vi "Write Abstract Message Definitions.vi"(10 "Abstract Message Definitions":T1, 11 "SCADA in":refnum<class "SCADA.lvclass">) -> (3 "SCADA out":refnum<class "SCADA.lvclass">)   [LabVIEW 2015, in "SCADA Core.lvlib" / "SCADA.lvclass"]
uses:
  SCADA.lvclass
  Controls/Abstract Messages Definitions Cluster.ctl
  SCADA Abstract Messages/Simple Command Status Msg/Simple Command Status Msg.lvclass
  SCADA Abstract Messages/IED Measurement Status Msg/IED Measurement Status Msg.lvclass
  SCADA Abstract Messages/Device Action Status Msg/Device Action Status Msg.lvclass
  SCADA Abstract Messages/Device Load Status Msg/Device Load Status Msg.lvclass
  SCADA Abstract Messages/IED Setpoint Status Msg/IED Setpoint Status Msg.lvclass
  SCADA Abstract Messages/Get Device Parameter Status Msg/Get Device Parameter Status Msg.lvclass
  SCADA Abstract Messages/Set Device Parameter Status Msg/Set Device Parameter Status Msg.lvclass
  SCADA Abstract Messages/Emergency Status Msg/Emergency Status Msg.lvclass
  SCADA Abstract Messages/Black Start Status Msg/Black Start Status Msg.lvclass
  SCADA Abstract Messages/Set Shed Sequence Status Msg/Set Shed Sequence Status Msg.lvclass
  SCADA.lvclass/SCADA.ctl
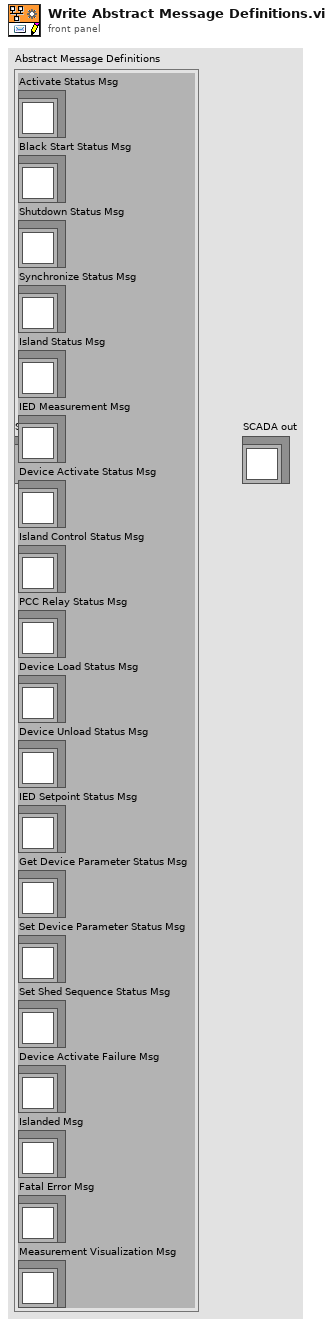
[diagram p1: front panel]
types:
  T1 = typedef "SCADA Core.lvlib/SCADA.lvclass/Abstract Messages Definitions Cluster.ctl" = cluster{"Activate Status Msg":refnum<class "Simple Command Status Msg.lvclass">, "Black Start Status Msg":refnum<class "Black Start Status Msg.lvclass">, "Shutdown Status Msg":refnum<class "Simple Command Status Msg.lvclass">, "Synchronize Status Msg":refnum<class "Simple Command Status Msg.lvclass">, "Island Status Msg":refnum<class "Simple Command Status Msg.lvclass">, "IED Measurement Msg":refnum<class "IED Measurement Status Msg.lvclass">, "Device Activate Status Msg":refnum<class "Device Action Status Msg.lvclass">, "Island Control Status Msg":refnum<class "Device Action Status Msg.lvclass">, "PCC Relay Status Msg":refnum<class "Device Action Status Msg.lvclass">, "Device Load Status Msg":refnum<class "Device Load Status Msg.lvclass">, "Device Unload Status Msg":refnum<class "Device Action Status Msg.lvclass">, "IED Setpoint Status Msg":refnum<class "IED Setpoint Status Msg.lvclass">, "Get Device Parameter Status Msg":refnum<class "Get Device Parameter Status Msg.lvclass">, "Set Device Parameter Status Msg":refnum<class "Set Device Parameter Status Msg.lvclass">, "Set Shed Sequence Status Msg":refnum<class "Set Shed Sequence Status Msg.lvclass">, "Device Activate Failure Msg":refnum<class "Emergency Status Msg.lvclass">, "Islanded Msg":refnum<class "Emergency Status Msg.lvclass">, "Fatal Error Msg":refnum<class "Emergency Status Msg.lvclass">, "Measurement Visualization Msg":refnum<class "IED Measurement Status Msg.lvclass">}
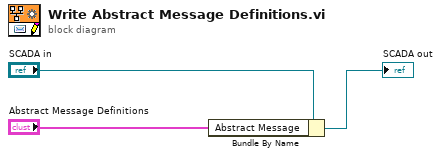
[diagram p0: block diagram]
diagram:
  n1 = Bundle By Name(cluster="SCADA in", "Abstract Message"="Abstract Message Definitions") -> (→"SCADA out":refnum<class "SCADA.lvclass">)
